vi "DatasocketsPart1.vi"() -> ()   [LabVIEW 2016]
uses:
  <vilib>/Utility/file.llb/Write Delimited Spreadsheet (DBL).vi
  <vilib>/Platform/browser.llb/Open URL in Default Browser (string).vi
panel:
  in  "?":bool
  out "See File":path
  out "Values Read":dbl[](array[numeric])
  in  "URL:":string="http://www.unm.edu/~mph/306/assignment6"
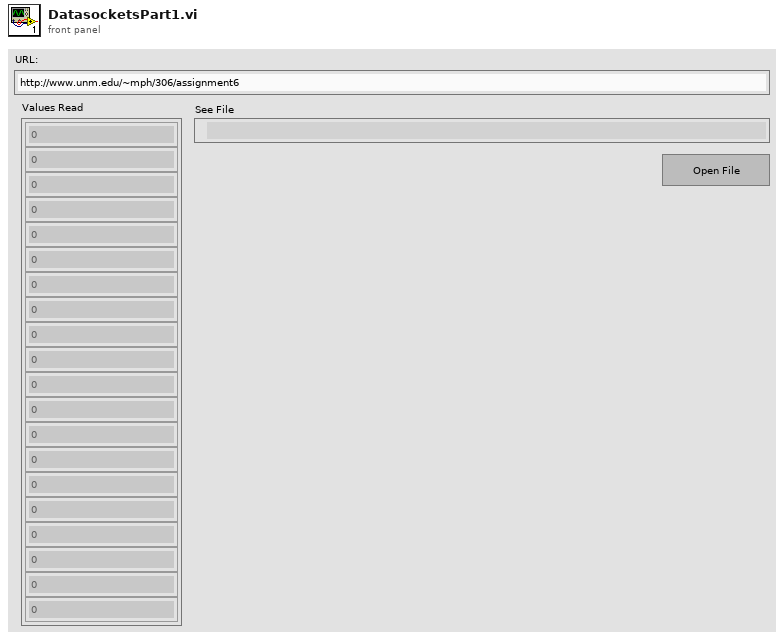
[diagram p1: front panel]
types:
  T1 = enum16{"Read", "Write", "ReadWrite", "BufferedRead", "BufferedReadWrite"}
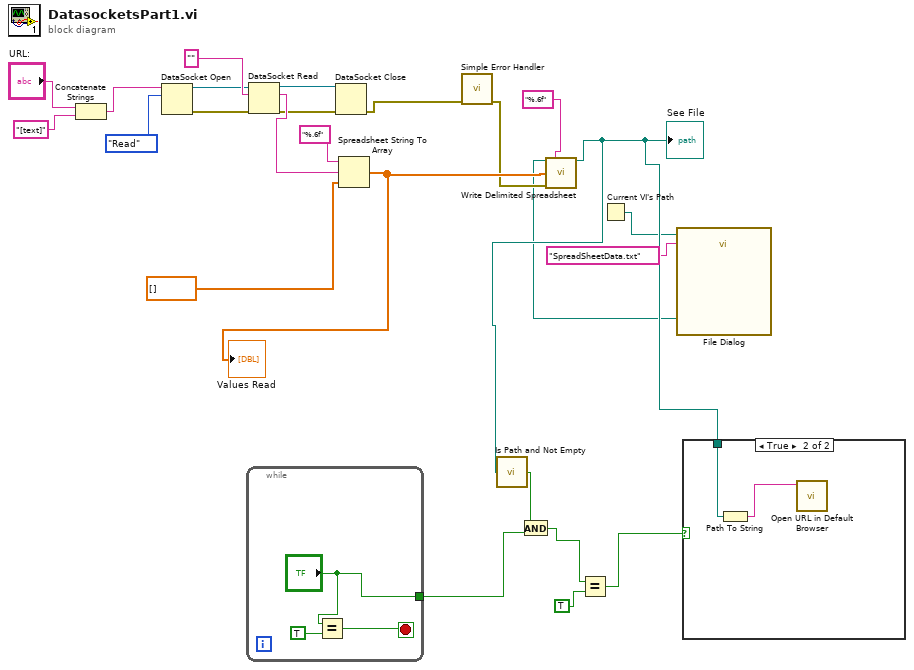
[diagram p0: block diagram]
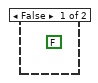
[diagram p2: hidden frame]
diagram:
  n1 = Concatenate Strings("URL:", "[text]" ("string")) -> (w17:string)
  n2 = DataSocket Open(10:T1."Read" ("mode"), 11:w17) -> (0:w13:errorcluster, 3:w14:refnum<k13>)  [unwired: 2 in]
  n3 = while {
    tunnel: ["?"] -> w25
    stop <- w26 stop-if-true
    n4 = Equal?(x="?", y=TRUE) -> (x = y?=w26:bool)
  }
  n5 = DataSocket Read(8:w13, 10:"", 11:w14) -> (0:w9:errorcluster, 2:w11:string, 3:w12:refnum<k13>)  [unwired: 2 in, 4 out]
  n6 = DataSocket Close(8:w9, 11:w12) -> (0:w5:errorcluster)  [unwired: 1 in, 1 out]
  n7 = Spreadsheet String To Array(format string="%.6f", spreadsheet string=w11, array type (2D Dbl)=dbl[] []) -> (array=w7:dbl[])  [unwired: 1 in]
  "Values Read" <- w7
  n8 = call <vilib>:"Simple Error Handler.vi"("error in (no error)"=w5) -> ("error out"=w4:errorcluster)  [unwired: 4 in, 4 out]
  n9 = Current VI's Path() -> (path=w1:path)
  n10 = call "File Dialog"("start path"=w1, "default name"="SpreadSheetData.txt") -> ("selected path"=w3:path)  [unwired: 10 in, 3 out]
  n11 = call-poly <vilib>:"Write Delimited Spreadsheet.vi"("file path (dialog if empty)"=w3, "format (%.3f)"="%.6f" ("format string"), "1D data"=w7, "error in (no error)"=w4) -> ("new file path (Not A Path if cancelled)"=w21:path)  [unwired: 10 in, 1 out]
  "See File" <- w21
  n12 = call <vilib>:"Is Path and Not Empty.vi"("path"=w21) -> ("Is Path and Not Empty?"=w20:bool)  [unwired: 4 in]
  n13 = And(x=w20, y=w25) -> (x .and. y?=w24:bool)
  n14 = Equal?(x=w24, y=TRUE) -> (x = y?=w22:bool)
  n15 = case shown="True" w22 {
    tunnel: w21 -> [_ w29]
    frame False {
      (unwired) FALSE
    }
    frame True {
      n16 = Path To String(path=w29) -> (string=w30:string)
      n17 = call-poly <vilib>:"Open URL in Default Browser.vi"("URL"=w30) -> ()  [unwired: 5 in, 2 out]
    }
  }
